vi "LVPortSetProperty.vi"(8 "Error in":errorcluster, 9 "Skip Parent Name (f)":bool, 10 "Value":variant, 11 "pID":string) -> (0 "Error out":errorcluster, 3 "Object map":T1[](array[typedef]))   [LabVIEW 2017]
uses:
  Common/ObjectMap/LVPortObjectMapNamepathData.ctl
  Common/ObjectMap/LVPortObjectMapDataTypeEnum.ctl
  Common/ObjectMap/LVPortObjectMapContainerTypeEnum.ctl
  Common/ObjectMap/LVPortObjectMapDefaultIDsEnum.ctl
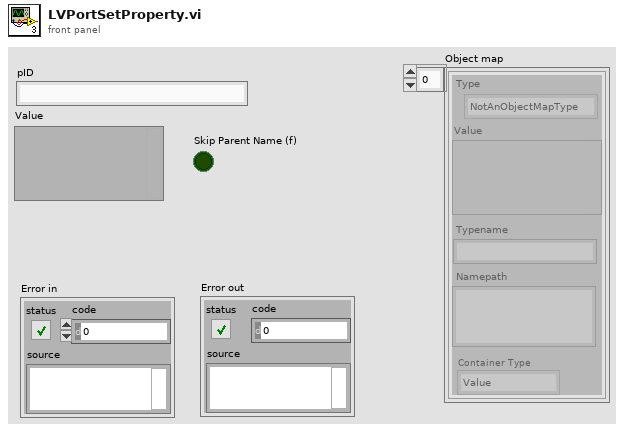
[diagram p1: front panel]
types:
  T1 = typedef "LVPortObjectMapNamepathData.ctl" = cluster{"Type":T2, "Value":variant, "Namepath":string, "Typename":string, "Container Type":T3}
  T2 = typedef "LVPortObjectMapDataTypeEnum.ctl" = enum16{"NotAnObjectMapType", "Real", "Complex", "String", "Boolean"}
  T3 = typedef "LVPortObjectMapContainerTypeEnum.ctl" = enum16{"Value", "Array", "Waveform"}
  T4 = typedef "LVPortObjectMapDefaultIDsEnum.ctl" = i32
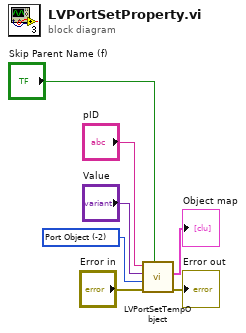
[diagram p0: block diagram]
diagram:
  w7 = T4 -2 items=["No ID"=-1, "Port Object"=-2] ("Default IDs")
  n1 = call "LVPortSetTempObject.vi"("Skip Parent Name"="Skip Parent Name (f)", "Error in"="Error in", "ID (-1 = new temp)"=w7, "Value"="Value", "pID"="pID") -> ("Error out"=→"Error out":errorcluster, "Object map"=→"Object map":T1[])  [unwired: 4 in, 1 out]
